vi "时间-温度曲线(子VI).vi"   [LabVIEW 2016, in "斯坦道CODMn新电路板.lvlib"]
uses:
  <vilib>/ptbypt/NI_PtbyPt.lvlib
types:
  T1 = enum16{"空闲", "水样测试", "标样核查", "零点核查", "跨度核查", "空白测试", "平行样测试", "加标回收", "空白校准", "标样校准", "初始化（清洗）"}
  T2 = cluster{"系统时间":timestamp, "工作状态":u16, "测量模式":enum16{"待机", "连续模式", "周期模式", "定点模式", "受控模式", "手动模式"}, "告警代码":u16, "故障代码":u16, "日志代码":u16, "软件版本":u16, "A":sgl, "B":sgl, "K":sgl, "当前滴定数":sgl, "T":sgl, "H":sgl, "id":u16, "flowid":u16, "量程":u16, "加热实时温度":sgl, "当前ORP值":sgl, "运行时间":sgl, "当前步骤剩余时间":sgl, "结束滴定数":sgl, "注射泵保温温度":sgl, "匹配滴定数X0":u16, "X^2":sgl, "X":sgl, "B 2":sgl}
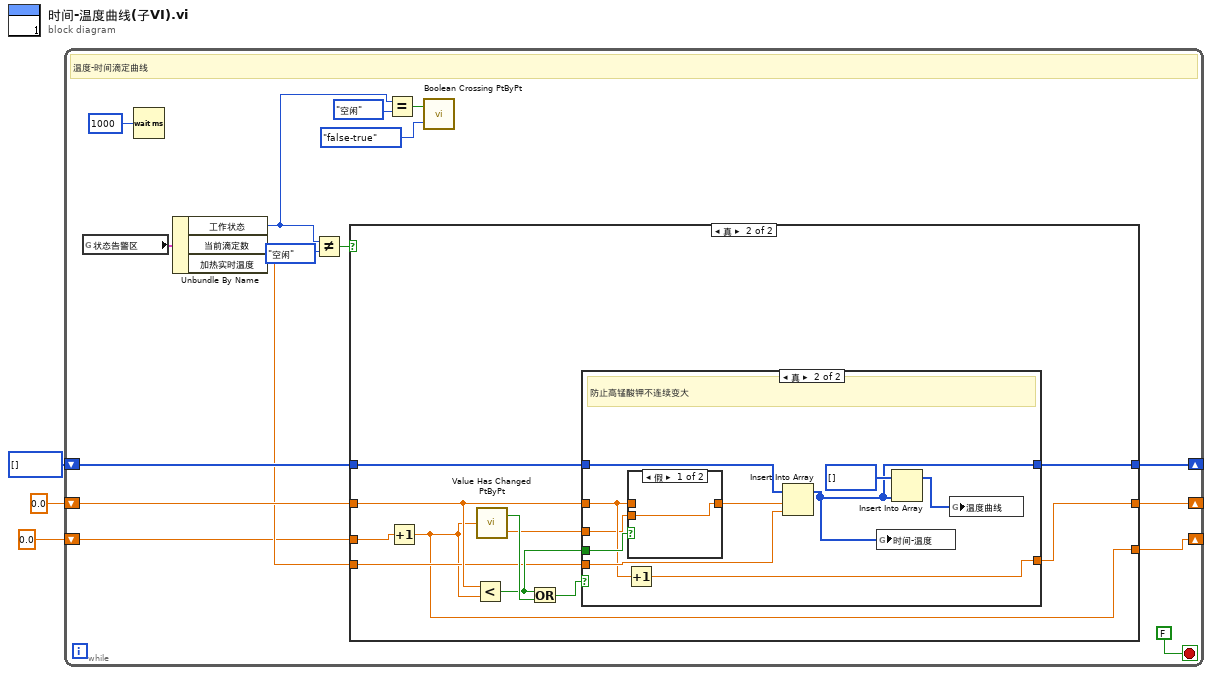
[diagram p0: block diagram]
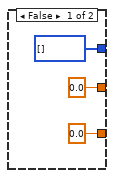
[diagram p2: hidden frame]
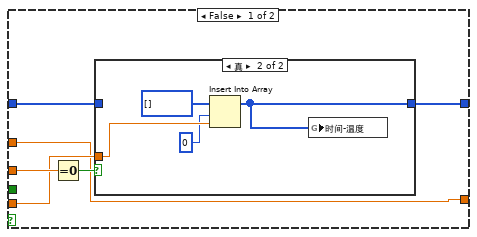
[diagram p3: hidden frame]
diagram:
  n1 = while {
    shift-right: [w16] -> _
    shift-left: u16[] [] ("ORP滴定曲线") -> [w17]
    shift-right: [w14] -> _
    shift-left: 0.0 -> [w15]
    shift-right: [w4] -> _
    shift-left: 0.0 -> [w5]
    stop <- FALSE stop-if-true
    # "温度-时间滴定曲线"
    n2 = global read "VARCODMn全局变量.vi" "状态告警区"() -> (w13:T2)
    n3 = Wait (ms)(milliseconds to wait=u32 1000 ("等待时间（毫秒）")) -> ()  [unwired: 1 out]
    n4 = Unbundle By Name(w13) -> ("工作状态"=w6:u16, "加热实时温度"=w10:sgl)  [unwired: 1 out]
    n5 = Not Equal?(x=w6, y=T1."空闲" ("工作状态")) -> (x != y?=w11:bool)
    n6 = case shown="真" w11 {
      tunnel: w17 -> [_ w33]
      tunnel: [u16[] [] ("ORP滴定曲线") w32] -> w16
      tunnel: w15 -> [_ w28]
      tunnel: [0.0 w27] -> w14
      tunnel: w10 -> [_ w25]
      tunnel: w5 -> [_ w24]
      tunnel: [0.0 w23] -> w4
      frame False {
      }
      frame True {
        n7 = Increment(x=w24) -> (x+1=w23:dbl)
        n8 = Less?(x=w28, y=w23) -> (x < y?=w26:bool)
        n9 = call <vilib>:"Value Has Changed PtByPt.vi"("input data point"=w23) -> ("has changed"=w31:bool, "output data point"=w30:dbl)  [unwired: 1 in]
        n10 = Or(x=w26, y=w31) -> (x .or. y?=w29:bool)
        n11 = case shown="真" w29 {
          tunnel: w33 -> [w38 w53]
          tunnel: [w37 w45] -> w32
          tunnel: w30 -> [w39 w47]
          tunnel: w25 -> [w35 w52]
          tunnel: w28 -> [w34 w49]
          tunnel: [w34 w51] -> w27
          tunnel: w26 -> [_ w50]
          frame False {
            n12 = Equal To 0?(x=w39) -> (x = 0?=w36:bool)
            n13 = case shown="真" w36 {
              tunnel: [w40 w41] -> w37
              tunnel: w38 -> [w40 _]
              tunnel: w35 -> [_ w43]
              frame False {
              }
              frame True {
                n14 = Insert Into Array(array=u16[] [] ("ORP滴定曲线"), index=0 ("索引"), new element=w43) -> (w41:u16[])
                n15 = global write "VARCODMn全局变量.vi" "时间-温度"(w41) -> ()
              }
            }
          }
          frame True {
            # "防止高锰酸钾不连续变大"
            n16 = Increment(x=w49) -> (x+1=w51:dbl)
            n17 = case shown="假" w50 {
              tunnel: w49 -> [_ w56]
              tunnel: [w55 w56] -> w48
              tunnel: w47 -> [w55 _]
              frame False {
              }
              frame True {
              }
            }
            n18 = Insert Into Array(array=w53, index=w48, new element=w52) -> (w45:u16[])
            n19 = global write "VARCODMn全局变量.vi" "时间-温度"(w45) -> ()
            n20 = Insert Into Array(array=u16[] [] ("ORP滴定曲线"), new element=w45) -> (w46:u16[])  [unwired: 1 in]
            n21 = global write "VARCODMn全局变量.vi" "温度曲线"(w46) -> ()
          }
        }
      }
    }
    n22 = Equal?(x=w6, y=T1."空闲" ("工作状态")) -> (x = y?=w8:bool)
    n23 = call <vilib>:"Boolean Crossing PtByPt.vi"("direction"=enum16{"either", "false-true", "true-false"}."false-true", "input"=w8) -> ()  [unwired: 1 in, 1 out]
  }
